vi "Read Units.vi"(8 "error in (no error)":errorcluster, 11 "9213 in":refnum<class "9212.lvclass">) -> (0 "error out":errorcluster, 2 "Units":T1[](array[typedef]) items=["Raw Volts", "Degrees Kelvin", "Degrees Celsius", "Degrees Fahrenheit", "Degrees Rankine"], 3 "9213 out":refnum<class "9212.lvclass">)   [LabVIEW 2014, in "Modules.lvlib" / "9212.lvclass"]
uses:
  9212.lvclass
  Measurement Units.ctl
  9212.lvclass/9212.ctl
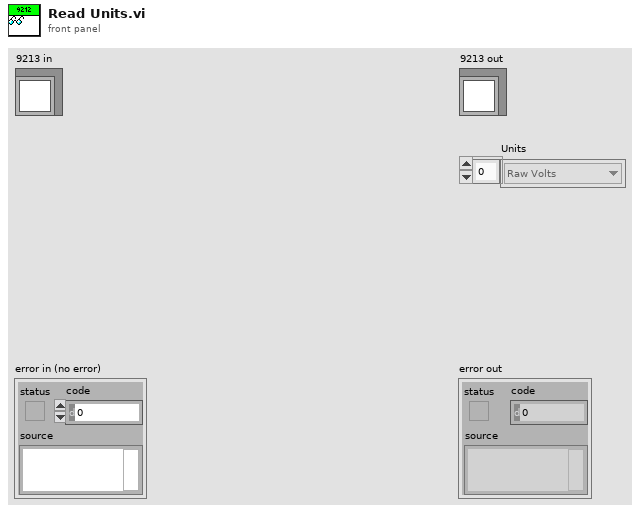
[diagram p1: front panel]
types:
  T1 = typedef "Modules.lvlib/9212.lvclass/Measurement Units.ctl" = u8
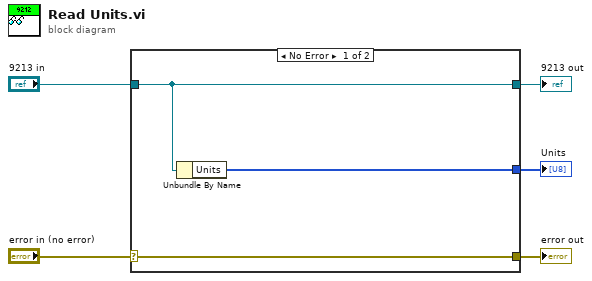
[diagram p0: block diagram]
diagram:
  n1 = case shown="No Error" "error in (no error)" {
    selector: "error in (no error)" -> [w8 w9]
    tunnel: [w8 w9] -> w4
    tunnel: [w7 w10] -> w2
    tunnel: "9213 in" -> [w7 w10]
    tunnel: [w6 _] -> w1
    frame No Error {
      n2 = Unbundle By Name(w7) -> ("Units"=w6:T1[])
    }
    frame Error {
    }
  }
  "error out" <- w4
  "9213 out" <- w2
  "Units" <- w1
